vi "ManipIntake.vi"(3 "Instruction String":string) -> (0 "Error Out":errorcluster, 1 "Advance Trigger":bool)   [LabVIEW 2020]
doc: "Toggles the intake deployment state.\n\nParameters: None"
uses:
  SafeParser_String.vi
  autonomousinfo.vi
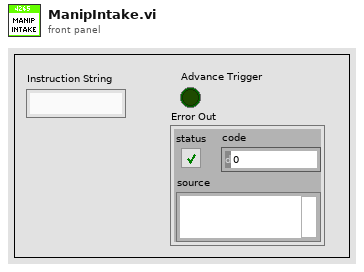
[diagram p1: front panel]
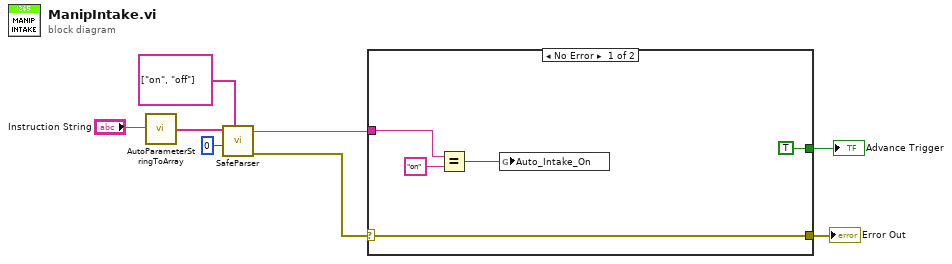
[diagram p0: block diagram]
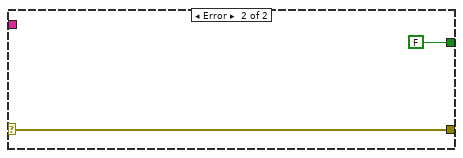
[diagram p2: hidden frame]
diagram:
  n1 = call "AutoParameterStringToArray.vi"("Parameter String"="Instruction String") -> ("Parsed Parameters"=w8:string[])
  n2 = call-poly "SafeParser.vi"("Allowed Values"=string[] ["on", "off"], "Array Index"=0 ("Parameter Index"), "String Array"=w8) -> ("Error Out"=w6:errorcluster, "Typecast Value"=w7:string)  [unwired: 7 in]
  n3 = case shown="No Error" w6 {
    selector: w6 -> [w12 w14]
    tunnel: [TRUE ("Advance Trigger") FALSE ("Advance Trigger")] -> w3
    tunnel: [w12 w14] -> w2
    tunnel: w7 -> [w11 _]
    frame No Error {
      n4 = Equal?(x=w11, y="on") -> (x = y?=w9:bool)
      n5 = global write "autonomousinfo.vi" "Auto_Intake_On"(w9) -> ()
    }
    frame Error {
    }
  }
  "Advance Trigger" <- w3
  "Error Out" <- w2
